vi "Run Filter.vi"(8 "error in (no error)":errorcluster, 10 "resource entries in":T1[](array[typedef]) {"FPGA CD Ref" format="%.0x"; "reserver" format="%.0x"}, 11 "And Filter in":refnum<class "AND Filter.lvclass">) -> (0 "error out":errorcluster, 2 "resource entries out":T1[](array[typedef]) {"FPGA CD Ref" format="%.0x"; "reserver" format="%.0x"})   [LabVIEW 2016, in "FPGA Resource Manager.lvlib" / "AND Filter.lvclass"]
uses:
  AND Filter/AND Filter.lvclass
  resource info.ctl
  <vilib>/NI Veristand/Custom Device API/Custom Device Item Ref.ctl
  AND Filter/AND Filter.lvclass/AND Filter.ctl
  Filter Parent/Filter.lvclass
  <vilib>/NI VeriStand/Custom Device API/Custom Device API.lvlib
  FPGA Resource Manager.lvlib
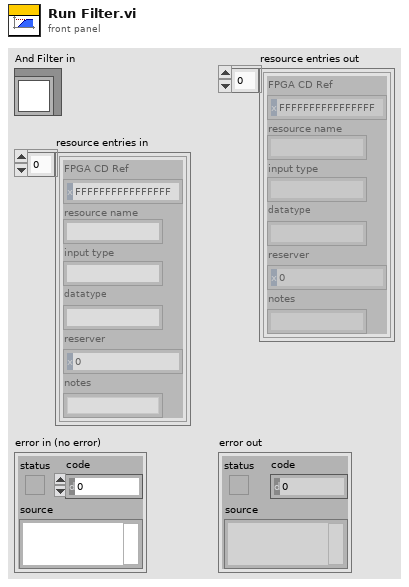
[diagram p1: front panel]
types:
  T1 = typedef "FPGA Resource Manager.lvlib/resource info.ctl" = cluster{"FPGA CD Ref":T2, "resource name":string, "input type":string, "datatype":string, "reserver":T2, "notes":string}
  T2 = typedef "Custom Device API.lvlib/Custom Device Item Ref.ctl" = u64
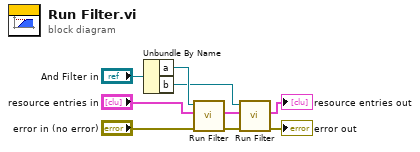
[diagram p0: block diagram]
diagram:
  n1 = Unbundle By Name("And Filter in") -> ("a"=w8:refnum<class "Filter.lvclass">, "b"=w6:refnum<class "Filter.lvclass">)
  n2 = call-dynamic "Run Filter.vi"("error in (no error)"="error in (no error)", "resource entries in"="resource entries in", "Filter in"=w8) -> ("error out"=w4:errorcluster, "resource entries out"=w5:T1[])  [unwired: 7 in]
  n3 = call-dynamic "Run Filter.vi"("error in (no error)"=w4, "resource entries in"=w5, "Filter in"=w6) -> ("error out"=→"error out":errorcluster, "resource entries out"=→"resource entries out":T1[])  [unwired: 7 in]
